vi "Assert Convert Time To Hour_Min.vi"() -> ()   [LabVIEW 2015, in "ExceelDate.lvclass"]
uses:
  ExceelDate.lvclass
panel:
  out "Hour:Min(\"\")":string
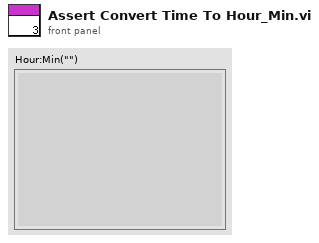
[diagram p1: front panel]
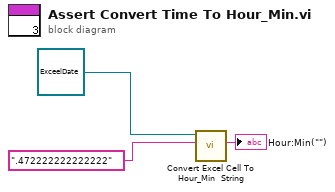
[diagram p0: block diagram]
diagram:
  n1 = call "Convert Excel Cell To Hour_Min  String.vi"("Hour:Min(\"\")"=".472222222222222" ("Hour:Min(\"\")"), "ExceelDate in"=refnum<class "ExceelDate.lvclass"> refnum) -> ("Hour:Min(\"\")"=→"Hour:Min(\"\")":string)  [unwired: 7 in, 2 out]
